vi "MaxVelocityConstraint_New.vi"(11 "Maximum Velocity":dbl format="%20.4f") -> (3 "MAX_VELOCITY_CONSTRAINT":T1 {"Max Velocity" format="%20.4f"})   [LabVIEW 2019, in "Trajectory_Library.lvlib"]
doc: "Constructs a maximum velocity constraint.\n\nParameters:\n - MaxVelocity - Maximum velocity\n\nReturns\n - MaxVelocityConstraint - Constraint data structure."
uses:
  Trajectory_Library.lvlib
  TypeDef/TRAJ_CONSTRAINT_MAX_VELOCITY.ctl
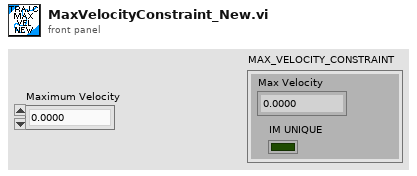
[diagram p1: front panel]
types:
  T1 = typedef "Trajectory_Library.lvlib/TRAJ_CONSTRAINT_MAX_VELOCITY.ctl" = cluster{"Max Velocity":dbl, "IM UNIQUE":bool}
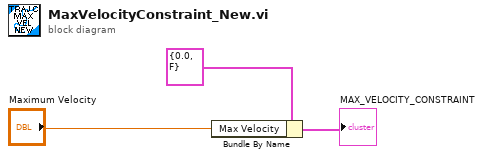
[diagram p0: block diagram]
diagram:
  n1 = Bundle By Name(cluster=T1 {"Max Velocity"=0.0, "IM UNIQUE"=FALSE} ("MAX_VELOCITY_CONSTRAINT"), "Max Velocity"="Maximum Velocity") -> (→"MAX_VELOCITY_CONSTRAINT":T1)
